vi "Debuging Indicator.vi"() -> (0 "String":string)   [LabVIEW 2014]
uses:
  <vilib>/Rock Robotics/Network Tables/SD Read Number.vi
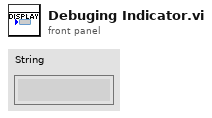
[diagram p1: front panel]
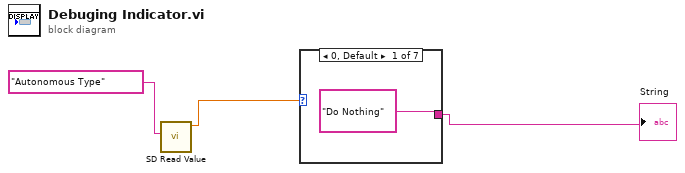
[diagram p0: block diagram]
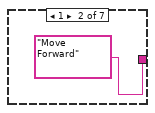
[diagram p2: hidden frame]
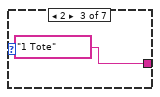
[diagram p3: hidden frame]
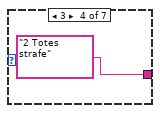
[diagram p4: hidden frame]
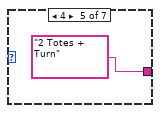
[diagram p5: hidden frame]
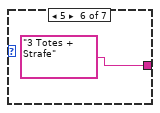
[diagram p6: hidden frame]
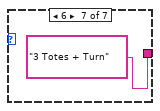
[diagram p7: hidden frame]
diagram:
  n1 = call-poly <vilib>:"SD Read Value.vi"("Table Prefix"="Autonomous Type" ("Name")) -> ("Numeric"=w2:dbl)  [unwired: 8 in, 2 out]
  n2 = case shown="0, Default" w2 {
    tunnel: ["Do Nothing" "Move Forward" "1 Tote" "2 Totes strafe" "2 Totes + Turn" "3 Totes + Strafe" "3 Totes + Turn"] -> w1
    frame 0, Default {
    }
    frame 1 {
    }
    frame 2 {
    }
    frame 3 {
    }
    frame 4 {
    }
    frame 5 {
    }
    frame 6 {
    }
  }
  "String" <- w1
